vi "Header Footer column.vi"(0 "Page points":T3={"Start at page"=612, "Page Size"=1, "Orientation"=enum."Landscape", "widht"=70.86614, "height"=70.86614, "Margin left"=70.86614, "Margin right"=72.0, "Margin top"=72.0, "Margin bottom"=72.0, "X0"=0.0, "X1"=612.0, "Y0"=0.0, "Y1"=792.0} {"Page Size" items=["Custom", "LETTER", "NOTE", "LEGAL", "TABLOID", "EXECUTIVE", "POSTCARD", "A0", "A1", "A2", "A3", "A4", "A5", "A6", "A7", "A8", "A9", "A10", "B0", "B1", "B2", "B3", "B4", "B5", "B6", "B7", "B8", "B9", "B10", "ARCH_E", "ARCH_D", "ARCH_C", "ARCH_B", "ARCH_A", "FLSA", "FLSE", "HALFLETTER", "_11X17", "ID_1", "ID_2", "ID_3", "LEDGER", "CROWN_QUARTO", "LARGE_CROWN_QUARTO", "DEMY_QUARTO", "ROYAL_QUARTO", "CROWN_OCTAVO", "LARGE_CROWN_OCTAVO", "DEMY_OCTAVO", "ROYAL_OCTAVO", "SMALL_PAPERBACK", "PENGUIN_SMALL_PAPERBACK", "PENGUIN_LARGE_PAPERBACK"]}, 1 "Header or Footer":T2, 7 "Table position IN":T1, 9 "numColumns":i32, 11 "error in (no error)":errorcluster) -> (8 "Table position OUT":T1, 10 "Table Column":dbl[](array[numeric]), 15 "error out":errorcluster)   [LabVIEW 2019]
doc: "Version 1.0\nDeveloped by Jean-Marc Simard\nCopyright © 2010, Exaprom Inc.\nAll rights reserved.\nLicense: BSD\n\nWith iTextSharp 4.1.6 (http://itextsharp.sourceforge.net)\nunder Mozilla Public License Version 1.1\n(http://www.mozilla.org/MPL/MPL-1.1.html)"
uses:
  <userlib>/Exaprom PDF/Controls/Page Controls/Page dimensions.ctl
  <userlib>/Exaprom PDF/Controls/Page Controls/Page size.ctl
  <userlib>/Exaprom PDF/Controls/Page Controls/Page Orientation.ctl
  <userlib>/Exaprom PDF/Controls/Header, Footer and Watermark Controls/Header or Footer.ctl
  <userlib>/Exaprom PDF/Controls/Header, Footer and Watermark Controls/Header or Footer Position.ctl
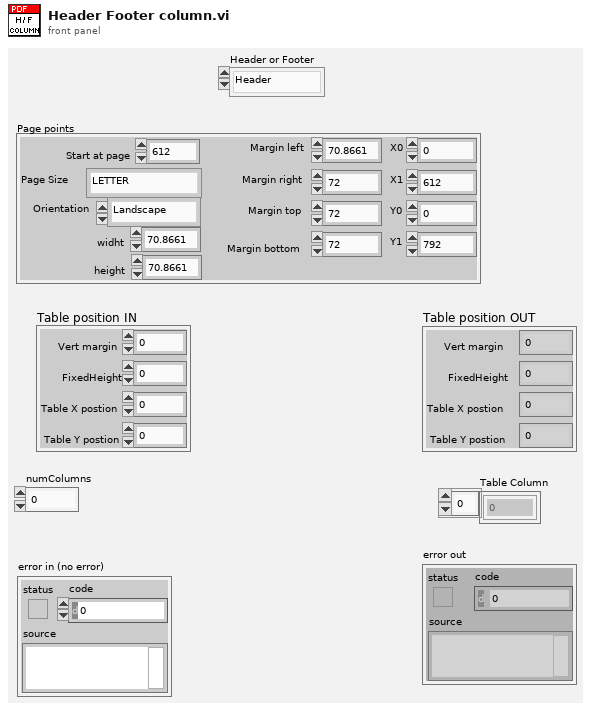
[diagram p1: front panel]
types:
  T1 = typedef "Header or Footer Position.ctl" = cluster{"Vert margin":dbl, "FixedHeight":dbl, "Table X postion":dbl, "Table Y postion":dbl}
  T2 = typedef "Header or Footer.ctl" = enum16{"Header", "Footer"}
  T3 = typedef "Page dimensions.ctl" = cluster{"Start at page":i32, "Page Size":T4, "Orientation":T5, "widht":sgl, "height":sgl, "Margin left":sgl, "Margin right":sgl, "Margin top":sgl, "Margin bottom":sgl, "X0":sgl, "X1":sgl, "Y0":sgl, "Y1":sgl}
  T4 = typedef "Page size.ctl" = i32
  T5 = typedef "Page Orientation.ctl" = enum16{"Portrait", "Landscape"}
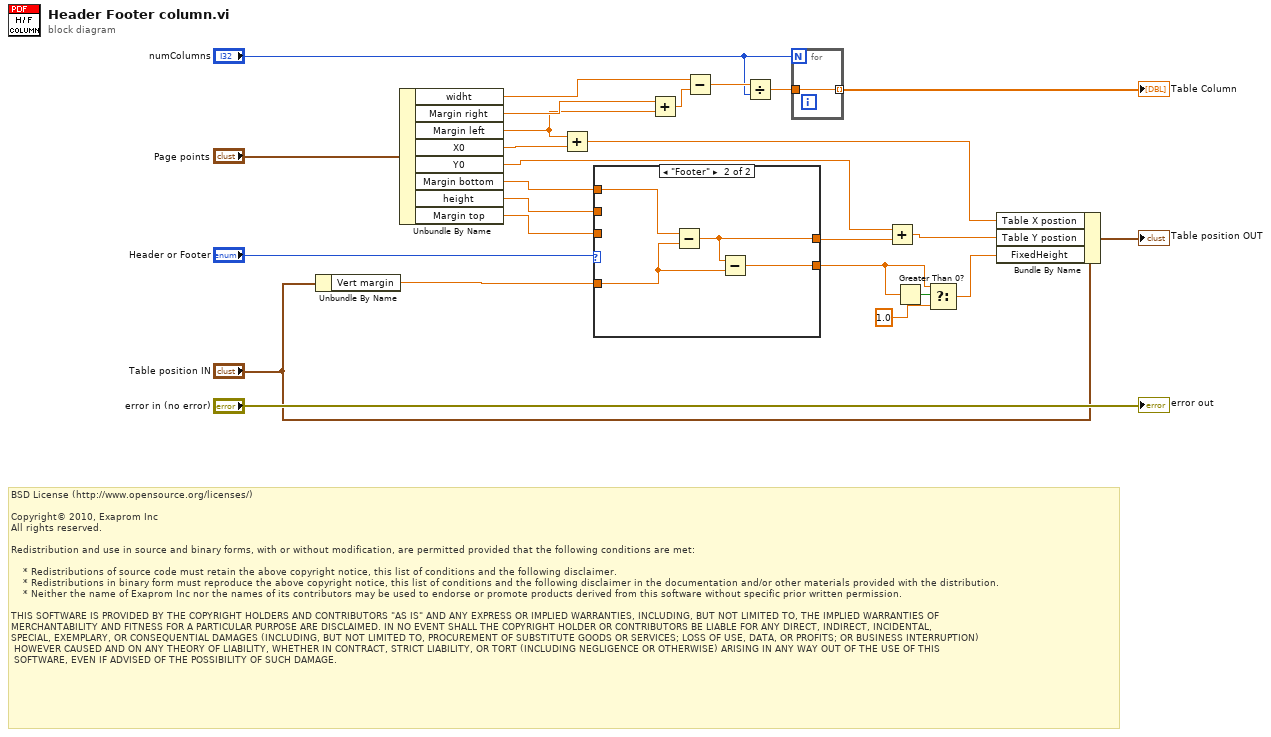
[diagram p0: block diagram]
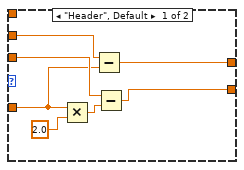
[diagram p2: hidden frame]
diagram:
  # "BSD License (http://www.opensource.org/licenses/)\n\nCopyright© 2010, Exaprom Inc\nAll rights reserved.\n\nRedistribution and use in source and binary forms, with or without modification, are permitted provided that the following conditions are met:\n\n    * Redistributions of source code must retain the above copyright notice, this list of conditions and the following disclaimer.\n    * Redistributions in binary form must reproduce the above copyright notice, this list of conditions and the following disclaimer in the documentation and/or other materials provided with the distribution.\n    * Neither the name of Exaprom Inc nor the names of its contributors may be used to endorse or promote products derived from this software without specific prior written permission.\n\nTHIS SOFTWARE IS PROVIDED BY THE COPYRIGHT HOLDERS AND CONTRIBUTORS \"AS IS\" AND ANY EXPRESS OR IMPLIED WARRANTIES, INCLUDING, BUT NOT LIMITED TO, THE IMPLIED WARRANTIES OF \nMERCHANTABILITY AND FITNESS FOR A PARTICULAR PURPOSE ARE DISCLAIMED. IN NO EVENT SHALL THE COPYRIGHT HOLDER OR CONTRIBUTORS BE LIABLE FOR ANY DIRECT, INDIRECT, INCIDENTAL,\nSPECIAL, EXEMPLARY, OR CONSEQUENTIAL DAMAGES (INCLUDING, BUT NOT LIMITED TO, PROCUREMENT OF SUBSTITUTE GOODS OR SERVICES; LOSS OF USE, DATA, OR PROFITS; OR BUSINESS INTERRUPTION)\n HOWEVER CAUSED AND ON ANY THEORY OF LIABILITY, WHETHER IN CONTRACT, STRICT LIABILITY, OR TORT (INCLUDING NEGLIGENCE OR OTHERWISE) ARISING IN ANY WAY OUT OF THE USE OF THIS\n SOFTWARE, EVEN IF ADVISED OF THE POSSIBILITY OF SUCH DAMAGE."
  n1 = Unbundle By Name("Table position IN") -> ("Vert margin"=w14:dbl)
  n2 = Unbundle By Name("Page points") -> ("widht"=w24:sgl, "Margin right"=w21:sgl, "Margin left"=w8:sgl, "X0"=w9:sgl, "Y0"=w1:sgl, "Margin bottom"=w4:sgl, "height"=w5:sgl, "Margin top"=w6:sgl)
  n3 = Add(x=w8, y=w9) -> (x+y=w7:sgl)
  n4 = case shown="\"Footer\"" "Header or Footer" {
    tunnel: w4 -> [_ w37]
    tunnel: w14 -> [w29 w35]
    tunnel: [w32 w36] -> w3
    tunnel: w5 -> [w33 _]
    tunnel: w6 -> [w31 _]
    tunnel: [w27 w34] -> w11
    frame "Header", Default {
      n5 = Multiply(x=w29, y=sgl 2.0) -> (x*y=w30:dbl)
      n6 = Subtract(x=w33, y=w29) -> (x-y=w32:dbl)
      n7 = Subtract(x=w31, y=w30) -> (x-y=w27:dbl)
    }
    frame "Footer" {
      n8 = Subtract(x=w37, y=w35) -> (x-y=w36:dbl)
      n9 = Subtract(x=w36, y=w35) -> (x-y=w34:dbl)
    }
  }
  n10 = Add(x=w21, y=w8) -> (x+y=w26:sgl)
  n11 = Subtract(x=w24, y=w26) -> (x-y=w25:sgl)
  n12 = Divide(x=w25, y="numColumns") -> (x/y=w17:sgl)
  n13 = for {
    N: "numColumns" -> [_]
    tunnel: w17 -> [w38]
    tunnel: [w38] -> w16 mode=indexing
  }
  "Table Column" <- w16
  n14 = Add(x=w1, y=w3) -> (x+y=w2:dbl)
  n15 = Greater Than 0?(x=w11) -> (x > 0?=w13:bool)
  n16 = Select(t=w11, s=w13, f=1.0) -> (s? t:f=w10:dbl)
  n17 = Bundle By Name(cluster="Table position IN", "Table X postion"=w7, "Table Y postion"=w2, "FixedHeight"=w10) -> (→"Table position OUT":T1)
  "error out" <- "error in (no error)"
